vi "Set Report Font.vi"(0 "report in":refnum<class "NI_report.lvclass">, 1 "text color (unchanged)":u32(colorbox)=16777216, 2 "font settings source (VI Inputs)":u16(ring) items=["VI Inputs", "Font Dialog Box"], 5 "text options":T2, 9 "font settings":T3={"Charset (-1)"=-1, "Weight (-1)"=-1, "Name"="", "Size"=" "}, 11 "error in (no error)":errorcluster) -> (4 "report out":refnum<class "NI_report.lvclass">, 6 "font out":T1={"font name"="", "font size"=0.0, "bold"=0, "italic"=0, "underline"=0, "strike through"=0, "font color"=16777216} {"font size" format="%0.2f"; "strike through" items=["Unchanged", "Yes", "No"]; "underline" items=["Unchanged", "Yes", "No"]; "italic" items=["Unchanged", "Yes", "No"]; "bold" items=["Unchanged", "Yes", "No"]}, 15 "error out":errorcluster)   [LabVIEW 2017, in "NI_report.lvclass"]
doc: "Sets the font properties of the report, including those in the headers and footers."
uses:
  <vilib>/Utility/NIReport.llb/NI_report.lvclass
  <vilib>/Utility/NIReport.llb/font.ctl
  <vilib>/Utility/NIReport.llb/NI_ReportGenerationCore.lvlib
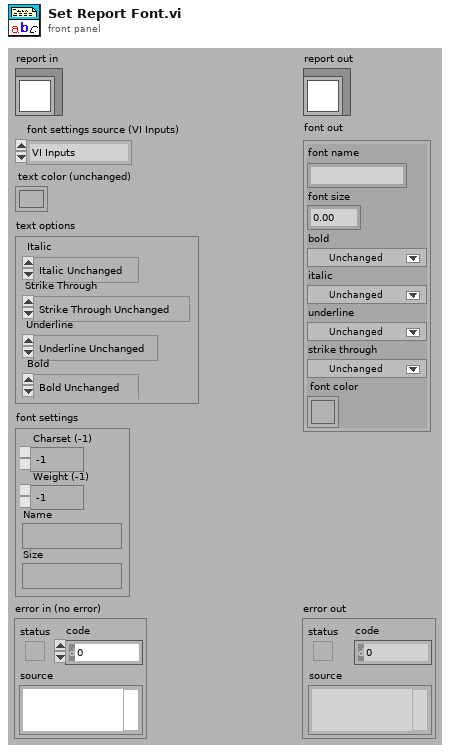
[diagram p1: front panel]
types:
  T1 = typedef "NI_ReportGenerationCore.lvlib/font.ctl" = cluster{"font name":string, "font size":dbl, "bold":u16, "italic":u16, "underline":u16, "strike through":u16, "font color":u32}
  T2 = cluster{"Italic":enum16{"Italic Unchanged", "Italic On", "Italic Off"}, "Strike Through":enum16{"Strike Through Unchanged", "Strike Through On", "Strike Through Off"}, "Underline":enum16{"Underline Unchanged", "Underline On", "Underline Off"}, "Bold":enum16{"Bold Unchanged", "Bold On", "Bold Off"}}
  T3 = cluster{"Charset (-1)":i16, "Weight (-1)":i16, "Name":string, "Size":string}
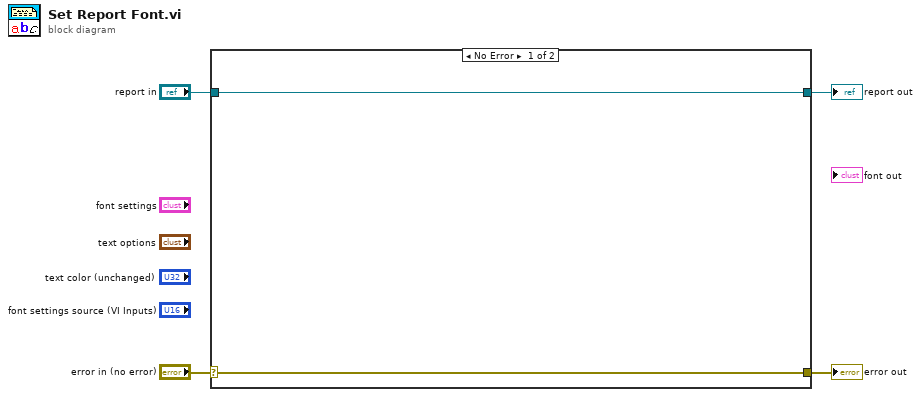
[diagram p0: block diagram]
diagram:
  n1 = case shown="No Error" "error in (no error)" {
    selector: "error in (no error)" -> [w5 w8]
    tunnel: [w5 w8] -> w3
    tunnel: [w6 w7] -> w1
    tunnel: "report in" -> [w6 w7]
    frame No Error {
    }
    frame Error {
    }
  }
  "error out" <- w3
  "report out" <- w1
